vi "AVPP_2_L6PAQ2hr.vi"(8 "error in (no error)":errorcluster, 9 "AverageAction IN":T1, 10 "PAQdatagram IN":T3 {"data" format="%.2f"; "status" format="%08x"}, 11 "AVPP in":refnum<class "AVPP.lvclass">) -> (0 "error out":errorcluster, 1 "Next_Level":T1, 3 "AVPP out":refnum<class "AVPP.lvclass">)   [LabVIEW 2014]
doc: "Process the Saving of 10 min samples towards the FAMM\n(into the 2 hrs buffer)"
uses:
  AVPP.lvclass
  HISW/controls/typedef_PAQdatagram.ctl
  FAMM/controls/typedef_AverageAction.ctl
  FAMM/controls/typedef_Level.ctl
  FAMM/controls/MemStoreDatagram.ctl
  FAMM/FAMM.lvclass
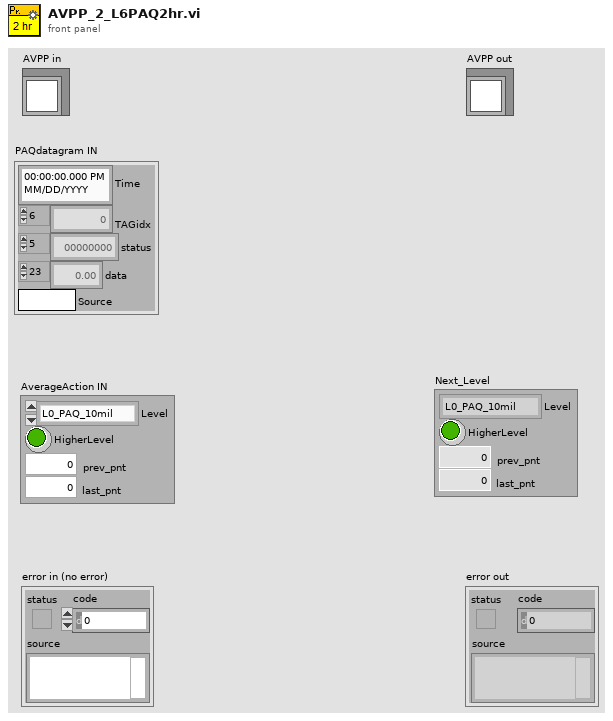
[diagram p1: front panel]
types:
  T1 = typedef "typedef_AverageAction.ctl" = cluster{"Level":T2, "HigherLevel":bool, "prev_pnt":i32, "last_pnt":i32}
  T2 = typedef "typedef_Level.ctl" = enum16{"L0_PAQ_10mil", "L0_PAQ_100mil", "L1_PAQ_100mil", "L2_PAQ_1sec", "L3_PAQ_10sec", "L4_PAQ_1min", "L5_PAQ_10min", "L6_PAQ_2hr", "L7_PAQ_1day", "L8_PAQ_1wk", "L1_PAQ_1sec", "L2_PAQ_10sec", "L3_PAQ_1min", "L4_PAQ_10min", "L5_PAQ_2hr", "L6_PAQ_1day", "L7_PAQ_1wk", "L0_PAQ_1sec", "L1_PAQ_10sec", "L2_PAQ_1min", "L3_PAQ_10min", "L4_PAQ_2hr", "L5_PAQ_1day", "L6_PAQ_1wk", "L0_PAQ_10sec", "L1_PAQ_1min", "L2_PAQ_10min", "L3_PAQ_2hr", "L4_PAQ_1day", "L5_PAQ_1wk"}
  T3 = typedef "typedef_PAQdatagram.ctl" = cluster{"Time":timestamp, "TAGidx":i32[], "status":u32[], "data":dbl[], "Source":string}
  T4 = typedef "FAMM.lvclass/MemStoreDatagram.ctl" = cluster{"Time":dbl, "TagIndex":i32[], "data":dbl[], "max":dbl[], "min":dbl[], "status":u32[], "Source":string}
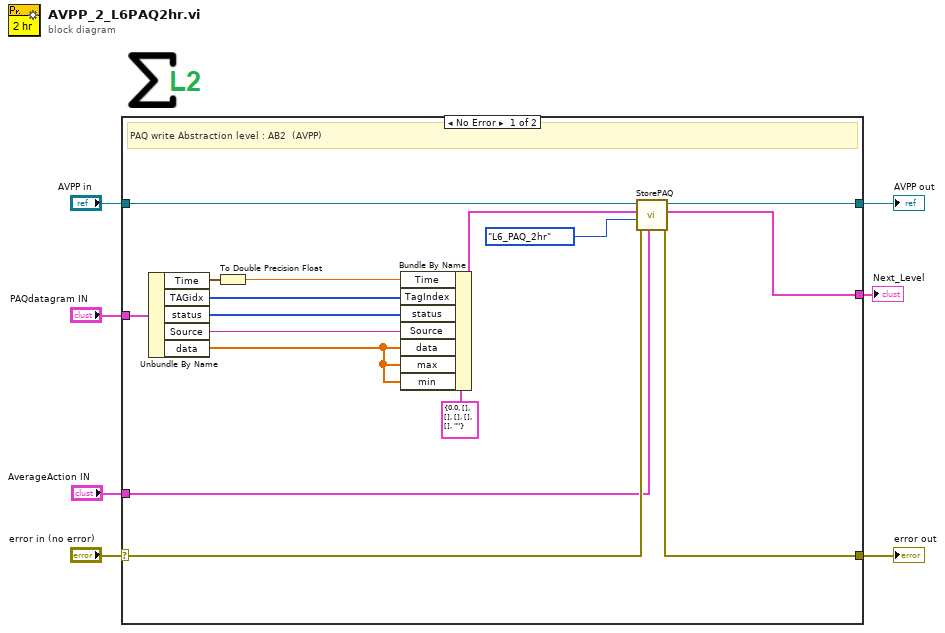
[diagram p0: block diagram]
diagram:
  n1 = case shown="No Error" "error in (no error)" {
    selector: "error in (no error)" -> [w12 w25]
    tunnel: [w11 w25] -> w6
    tunnel: [w23 w24] -> w4
    tunnel: "AVPP in" -> [w17 w24]
    tunnel: "PAQdatagram IN" -> [w21 _]
    tunnel: [w9 _] -> w2
    tunnel: "AverageAction IN" -> [w8 _]
    frame No Error {
      # "PAQ write Abstraction level : AB2  (AVPP)"
      n2 = Unbundle By Name(w21) -> ("Time"=w20:timestamp, "TAGidx"=w18:i32[], "status"=w16:u32[], "Source"=w15:string, "data"=w13:dbl[])
      n3 = To Double Precision Float(number=w20) -> (double precision float=w19:dbl)
      n4 = Bundle By Name(cluster=T4 {"Time"=0.0, "TagIndex"=[], "data"=[], "max"=[], "min"=[], "status"=[], "Source"=""} ("StoreDatagram"), "Time"=w19, "TagIndex"=w18, "status"=w16, "Source"=w15, "data"=w13, "max"=w13, "min"=w13) -> (w14:T4)
      n5 = call "StorePAQ.vi"("AverageAction IN"=w8, "error in (no error)"=w12, "Level"=typedef_Level."L6_PAQ_2hr" ("Enum"), "StoreDatagram"=w14, "FAMM in"=w17) -> ("error out"=w11:errorcluster, "Next_Level"=w9:T1, "FAMM out"=w23:refnum<class "AVPP.lvclass">)  [unwired: 4 in]
    }
    frame Error {
    }
  }
  "error out" <- w6
  "AVPP out" <- w4
  "Next_Level" <- w2
